vi "A_star.vi"(8 "Map":dbl[][](array[numeric]), 9 "Ed":cluster{"X":i32, "Y":i32}, 11 "St":cluster{"X":i32, "Y":i32}) -> (0 "Map_out":dbl[][](array[numeric]), 3 "Path":dbl[][](array[numeric]))   [LabVIEW 2017]
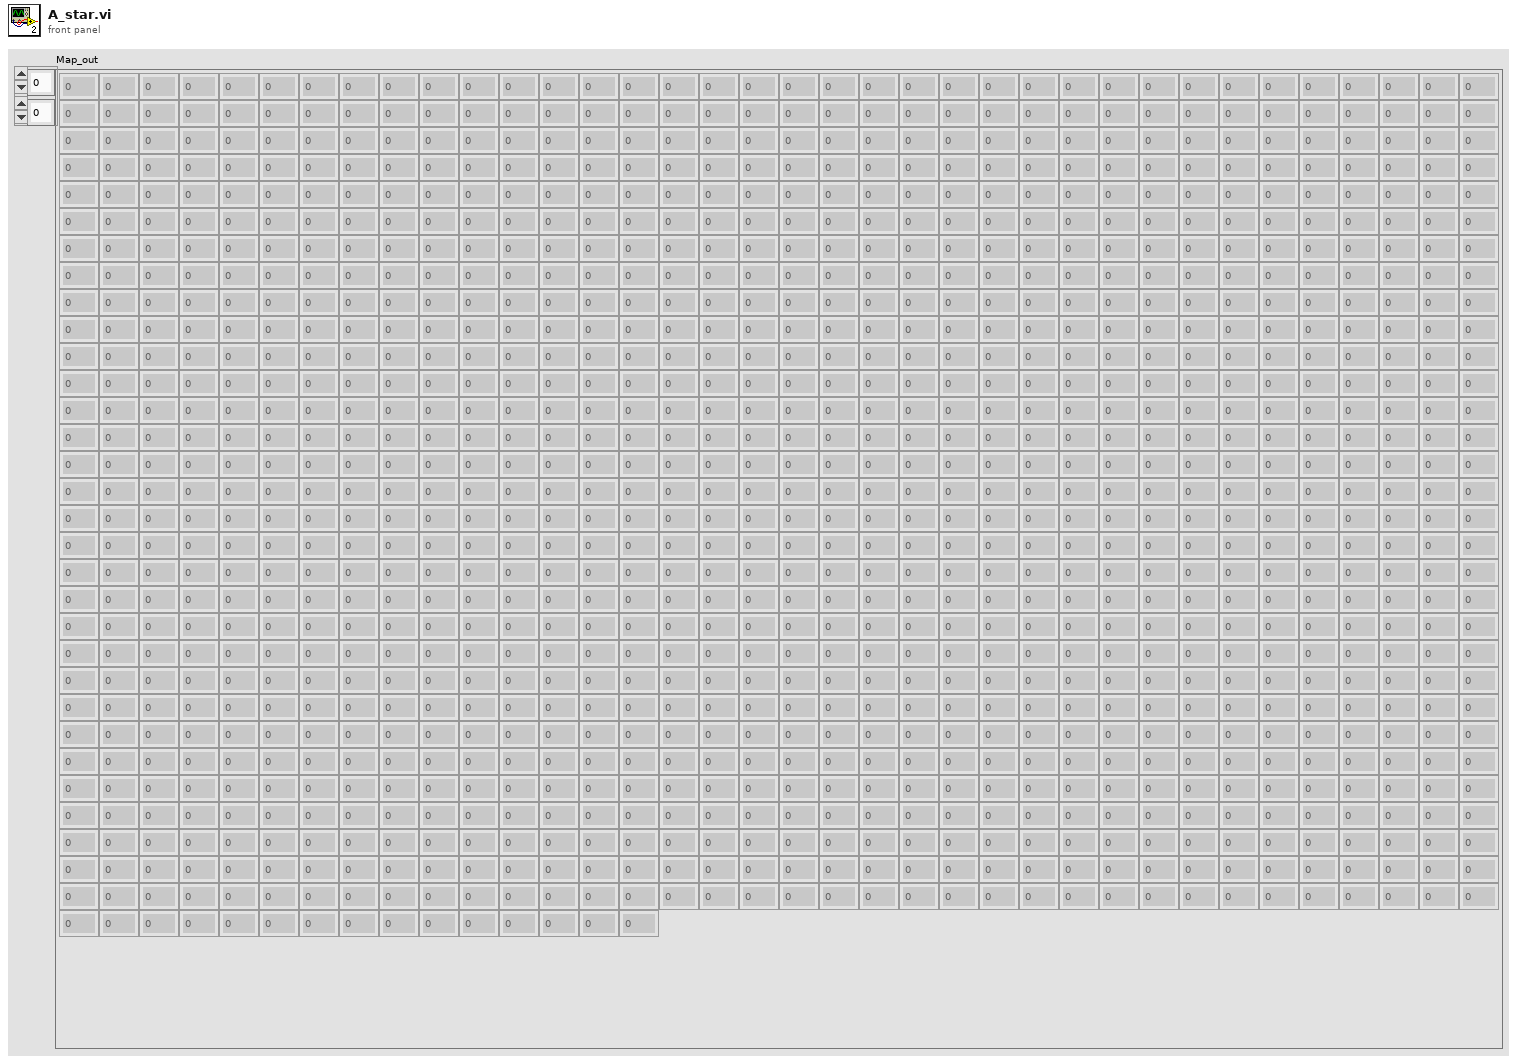
[diagram p1: front panel]
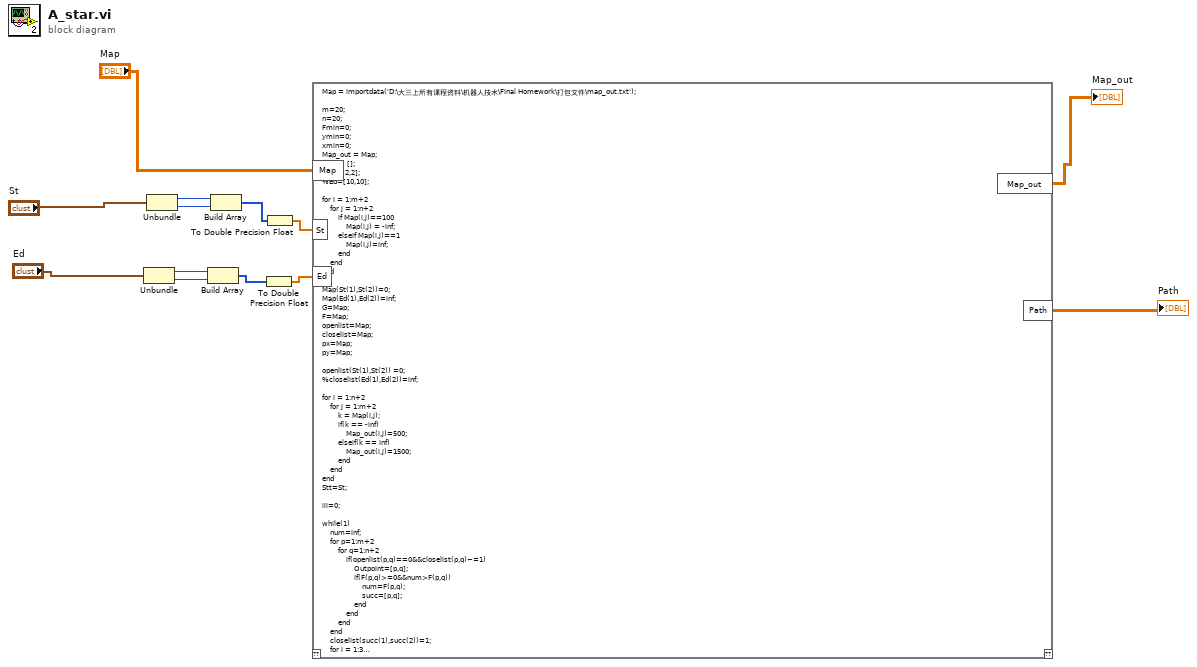
[diagram p0: block diagram]
diagram:
  n1 = Unbundle("Ed") -> ("X"=w10:i32, "Y"=w9:i32)
  n2 = Unbundle("St") -> ("X"=w12:i32, "Y"=w11:i32)
  n3 = Build Array(w10, w9) -> (w6:i32[])
  n4 = Build Array(w12, w11) -> (w8:i32[])
  n5 = To Double Precision Float(number=w6) -> (double precision float=w5:dbl[])
  n6 = To Double Precision Float(number=w8) -> (double precision float=w7:dbl[])
  n7 = script code="Map = importdata('D:\\大三上所有课程资料\\机器人技术\\Final Homework\\打包文件\\map_out.txt');\n\nm=20;\nn=20;\nFmin=0;\nymin=0;\nxmin=0;\nMap_out = Map;\nPath = [];\n%St=[2,2];\n%Ed=[10,10];\n\nfor i = 1:m+2\n    for j = 1:n+2\n        if Map(i,j)==100\n            Map(i,j) = -inf;\n        elseif Map(i,j)==1\n            Map(i,j)=inf;\n        end\n    end\nend\n\nMap(St(1),St(2))=0;\nMap(Ed(1),Ed(2))=inf;\nG=Map;\nF=Map;\nopenlist=Map;\ncloselist=Map;\npx=Map;\npy=Map;\n\nopenlist(St(1),St(2)) =0;\n%closelist(Ed(1),Ed(2))=inf;\n\nfor i = 1:n+2\n    for j = 1:m+2\n        k = Map(i,j);\n        if(k == -inf)\n            Map_out(i,j)=500;\n        elseif(k == inf)\n            Map_out(i,j)=1500;\n        end\n    end\nend\nStt=St;\n\niii=0;\n\nwhile(1)\n    num=inf;\n    for p=1:m+2\n        for q=1:n+2\n            if(openlist(p,q)==0&&closelist(p,q)~=1)\n                Outpoint=[p,q];\n                if(F(p,q)>=0&&num>F(p,q))\n                    num=F(p,q);\n                    succ=[p,q];\n                end\n            end\n        end\n    end\n    closelist(succ(1),succ(2))=1;\n    for i = 1:3\n        for j = 1:3\n            k = G(succ(1)-2+i,succ(2)-2+j);\n            if((i+j==4)|(i==j)|closelist(succ(1)-2+i,succ(2)-2+j)==1)\n                continue;  %遇见起点,已经过的点\n            elseif (k == -inf)\n                G(succ(1)-2+i,succ(2)-2+j) = G(succ(1)-2+i,succ(2)-2+j);\n                closelist(succ(1)-2+i,succ(2)-2+j)=1;  %遇见障碍\n            elseif (k == inf)\n                distance=abs(succ(1)-2+i-St(1))+abs(succ(2)-2+j-St(2)); \n                G(succ(1)-2+i,succ(2)-2+j)=G(succ(1),succ(2))+distance;   %加入距离\n                openlist(succ(1)-2+i,succ(2)-2+j)=0;                               %设置为待搜索节点\n\n%------------------------------------------------------估价函数H\n                  H_diagonal=abs(succ(1)-2+i-Ed(1));\n                  H_straight=abs(succ(2)-2+j-Ed(2));\n                  H=H_diagonal+H_straight;\n                \n                F(succ(1)-2+i,succ(2)-2+j)=G(succ(1)-2+i,succ(2)-2+j)+H;   %从起点到该处再到终点的总代价\n                px(succ(1)-2+i,succ(2)-2+j)=succ(1);\n                py(succ(1)-2+i,succ(2)-2+j)=succ(2);\n            else\n                 distance=abs(succ(1)-2+i-St(1))+abs(succ(2)-2+j-St(2));%更新节点信息情况\n                if(k>(distance+G(succ(1),succ(2))))\n                k=distance+G(succ(1),succ(2));\n\n%--------估价函数H\n                     H_diagonal=abs(succ(1)-2+i-Ed(1));\n                     H_straight=abs(succ(2)-2+j-Ed(2));\n                     H=H_diagonal+H_straight;\n                \n\n                F(succ(1)-2+i,succ(2)-2+j)=k+H;\n                px(succ(1)-2+i,succ(2)-2+j)=succ(1);\n                py(succ(1)-2+i,succ(2)-2+j)=succ(2);\n                end\n            end\n            if(((succ(1)-2+i)==Ed(1)&&(succ(2)-2+j)==Ed(2))|num==inf)\n                 px(Ed(1),Ed(2))=succ(1);\n                py(Ed(1),Ed(2))=succ(2);\n                break;\n            end\n        end\n        if(~((i+j==4)|(i==j))&&((succ(1)-2+i)==Ed(1)&&(succ(2)-2+j)==Ed(2))|num==inf)\n             px(Ed(1),Ed(2))=succ(1);\n                py(Ed(1),Ed(2))=succ(2);\n            break;\n        end\n    %------------\n        if((i==3)&&(j==3))\n            Fmin=F(succ(1)-1,succ(2));\n            xmin=succ(1)-1;\n            ymin=succ(2);\n            for w=1:3\n               for l=1:3\n                  if ((w+l==4)|(w==l))\n                      continue;\n                  elseif (F(succ(1)-2+w,succ(2)-2+l)<Fmin)\n                      Fmin=F(succ(1)-2+w,succ(2)-2+l);\n                      xmin=succ(1)-2+w;\n                      ymin=succ(2)-2+l;\n                  elseif (F(succ(1)-2+w,succ(2)-2+l)==Fmin)\n                      xearlier=px(succ(1),succ(2));\n                      yearlier=py(succ(1),succ(2));\n                      if ((abs(succ(2)-yearlier)==1)&&(abs(succ(1)-xearlier)==0))\n                          if(abs(succ(1)-2+w-succ(1))==0)\n                              closelist(xmin,ymin)=1;\n                          else closelist(succ(1)-2+w,succ(2)-2+l)=1;\n                          end\n                      elseif ((abs(succ(2)-yearlier)==0)&&(abs(succ(1)-xearlier)==1))\n                          if(abs(succ(2)-2+l-succ(2))==0)\n                          closelist(xmin,ymin)=1;\n                          else closelist(succ(1)-2+w,succ(2)-2+l)=1;\n                          end\n                      end\n                  end\n               end\n            end\n        end\n%-------------------------------\n   end\n    if(~((i+j==4)|(i==j))&&((succ(1)-2+i)==Ed(1)&&(succ(2)-2+j)==Ed(2))|num==inf)\n         px(Ed(1),Ed(2))=succ(1);\n                py(Ed(1),Ed(2))=succ(2);\n        break;\n    end\nend\n%------------------------------------------输出路径---------------------------------------------\n    P=[];\n    s=1;\nwhile(1)\n    if(num==inf)\n        break;\n    end\n    iii=iii+1;\n    Map_out(Ed(1),Ed(2))=iii;\n    Path(iii,1)=Ed(1);\n    Path(iii,2)=Ed(2);\n\n    P(s,:)=Ed;\n    s=s+1;\n%      pause(1);\n    xx=Ed(1);\n    Ed(1)=px(Ed(1),Ed(2));\n    Ed(2)=py(xx,Ed(2));\n    if(px(Ed(1),Ed(2))==St(1)&&py(Ed(1),Ed(2))==St(2))\n        iii=iii+1;\n        Map_out(Ed(1),Ed(2))=iii;\n        Path(iii,1)=Ed(1);\n        Path(iii,2)=Ed(2);\n        P(s,:)=Ed;\n        break;\n    end\nend\nP(s+1,:)=St;\n\niii=iii+1;\nMap_out(Stt(1),Stt(2))=iii;\nPath(iii,1)=Stt(1);\nPath(iii,2)=Stt(2);\n\ncnt=0;\nfor i=2:m\n    for j=2:n\n        if(G(i,j)~=inf&&G(i,j)~=-inf)\n            cnt=cnt+1;\n        end\n    end\nend"("Map"="Map", "St"=w7, "Ed"=w5) -> ("Map_out"=→"Map_out":dbl[][], "Path"=→"Path":dbl[][])  [unwired: 1 in, 1 out]
